vi "Merge.vi"(8 "error in (no error)":errorcluster, 9 "TTLDevice in 2":refnum<class "TTLControlledDevice.lvclass">, 11 "TTLDevice in":refnum<class "TTLControlledDevice.lvclass">) -> (0 "error out":errorcluster, 3 "TTLDevice out":refnum<class "TTLControlledDevice.lvclass">)   [LabVIEW 2015, in "TTLControlledDevice.lvclass"]
uses:
  TTLControlledDevice.lvclass
  TTLControlledDevice.lvclass/TTLControlledDevice.ctl
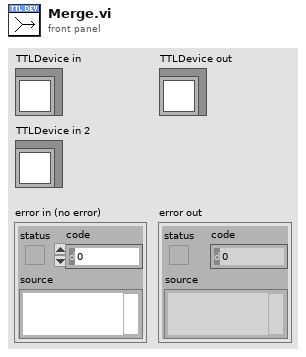
[diagram p1: front panel]
types:
  T1 = typedef "TTLControlledDevice.lvclass/Serialized.ctl" = cluster{"Name":string, "Line":string}
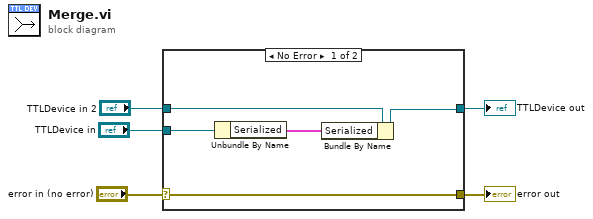
[diagram p0: block diagram]
diagram:
  n1 = case shown="No Error" "error in (no error)" {
    selector: "error in (no error)" -> [w10 w12]
    tunnel: [w10 w12] -> w4
    tunnel: [w9 w11] -> w2
    tunnel: "TTLDevice in" -> [w7 w11]
    tunnel: "TTLDevice in 2" -> [w6 _]
    frame No Error {
      n2 = Unbundle By Name(w7) -> ("Serialized"=w8:T1)
      n3 = Bundle By Name(cluster=w6, "Serialized"=w8) -> (w9:refnum<class "TTLControlledDevice.lvclass">)
    }
    frame Error {
    }
  }
  "error out" <- w4
  "TTLDevice out" <- w2
